vi "Test 2 Serial Write Data is Written to Decorated Interface.vi"(8 "error in (no error)":errorcluster, 11 "Serial Logging Decorator Test In":refnum<class "Serial Logging Decorator Test.lvclass">) -> (0 "error out":errorcluster, 3 "Serial Logging Decorator Test Out":refnum<class "Serial Logging Decorator Test.lvclass">)   [LabVIEW 2020, in "Serial Logging Decorator Test.lvclass"]
uses:
  Serial Logging Decorator Test.lvclass
  C:/Program Files (x86)/National Instruments/LabVIEW 2020/vi.lib/Astemes/LUnit/Test Case.lvclass
  Log/Log.lvclass
  Mock Serial/Mock Serial.lvclass
  C:/Program Files (x86)/National Instruments/LabVIEW 2020/vi.lib/Astemes/LMock/Mock.lvclass
  C:/git/astemes-lmock/sandbox/Examples/Serial/Serial.lvclass/Serial.lvclass
  <vilib>/Astemes/LMock/One Identical Inputs.vi
  Serial/Serial.lvclass/Serial.lvclass
  Serial Logging Decorator/Serial Logging Decorator.lvclass
  <vilib>/Astemes/LMock/LMock.lvlib
  <vilib>/Astemes/LMock/LMock Verifier.lvclass
  C:/git/astemes-lmock/sandbox/Examples/Mock Serial/Mock Serial.lvclass
  <vilib>/Astemes/LMock/LMock One.lvlib
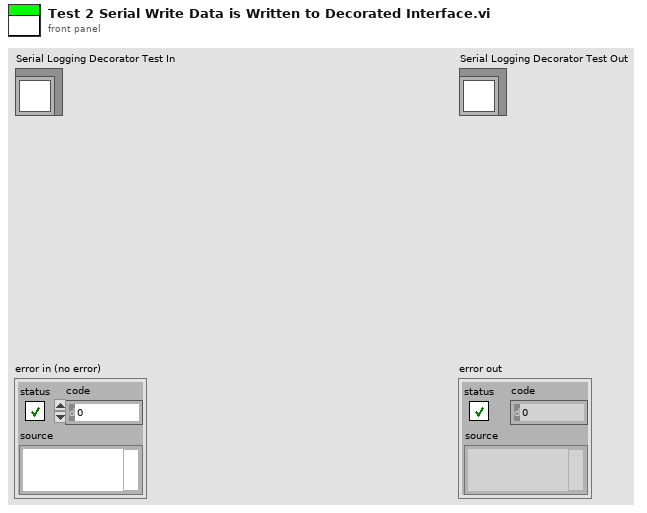
[diagram p1: front panel]
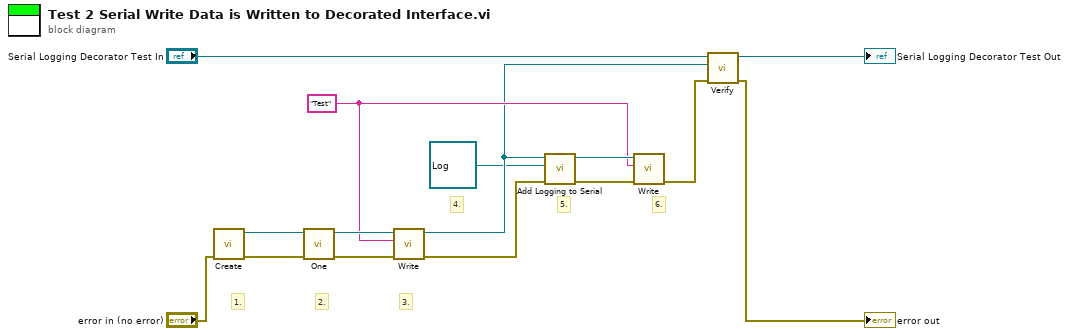
[diagram p0: block diagram]
diagram:
  w5 = "Test" ("Text to Write")
  # "6."
  # "5."
  # "4."
  # "3."
  # "2."
  # "1."
  n1 = call "Create.vi"("error in (no error)"="error in (no error)") -> ("error out"=w11:errorcluster, "Mock Class Generator out"=w12:refnum<class "Mock Serial.lvclass">)  [unwired: 9 in]
  n2 = call-poly <vilib>:"One.vi"("error in (no error)"=w11, "Mock in"=w12) -> ("error out"=w9:errorcluster, "Mock out"=w10:refnum<class "Mock Serial.lvclass">)  [unwired: 8 in]
  n3 = call-dynamic "Write.vi"("error in (no error)"=w9, "write buffer"=w5, "Serial in"=w10) -> ("error out"=w6:errorcluster, "Serial out"=w2:refnum<class "Mock Serial.lvclass">)  [unwired: 6 in, 1 out]
  n4 = call "Add Logging to Serial.vi"("error in (no error)"=w6, "Log Destination"=refnum<class "Log.lvclass"> refnum ("Log.lvclass"), "Serial"=w2) -> ("error out"=w7:errorcluster, "Serial with Logging"=w8:refnum<class "Serial.lvclass">)  [unwired: 7 in]
  n5 = call-dynamic "Write.vi"("error in (no error)"=w7, "write buffer"=w5, "Serial in"=w8) -> ("error out"=w3:errorcluster)  [unwired: 6 in, 2 out]
  n6 = call <vilib>:"Verify.vi"("error in (no error)"=w3, "Mock"=w2, "LUnit Test Case In"="Serial Logging Decorator Test In") -> ("error out"=→"error out":errorcluster, "LUnit Test Case Out"=→"Serial Logging Decorator Test Out":refnum<class "Serial Logging Decorator Test.lvclass">)  [unwired: 7 in]
